vi "Test_Get MetaData.vi"() -> ()   [LabVIEW 2020]
uses:
  Measurement_client/RPC Messages/ni_measurements_v1_GetMetadataResponse.ctl
  Measurement_client/RPC Messages/ni_measurements_v1_MeasurementDetails.ctl
  Measurement_client/RPC Messages/ni_measurements_v1_MeasurementParameters.ctl
  Measurement_client/RPC Messages/ni_measurements_v1_ConfigurationParameter.ctl
  Measurement_client/RPC Messages/google_protobuf_Any.ctl
  Measurement_client/RPC Messages/ni_measurements_v1_Output.ctl
  Measurement_client/RPC Messages/ni_measurements_v1_UserInterfaceDetails.ctl
  Measurement_client/RPC Messages/ni_measurements_v1_GetMetadataRequest.ctl
  Measurement_client/Measurement_client.lvlib
panel:
  out "Response Data":T1
  in  "address":string
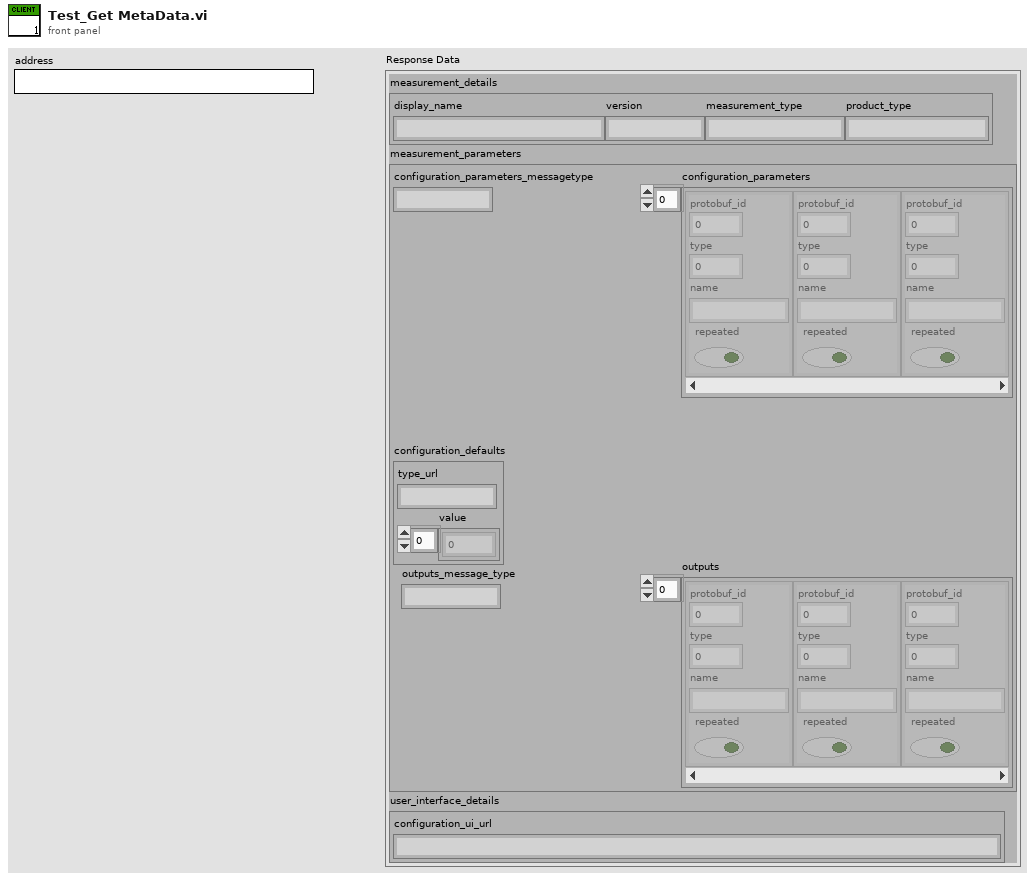
[diagram p1: front panel]
types:
  T1 = typedef "Measurement_client.lvlib/ni_measurements_v1_GetMetadataResponse.ctl" = cluster{"measurement_details":T2, "measurement_parameters":T3, "user_interface_details":T7}
  T2 = typedef "Measurement_client.lvlib/ni_measurements_v1_MeasurementDetails.ctl" = cluster{"display_name":string, "version":string, "measurement_type":string, "product_type":string}
  T3 = typedef "Measurement_client.lvlib/ni_measurements_v1_MeasurementParameters.ctl" = cluster{"configuration_parameters_messagetype":string, "configuration_parameters":T4[], "configuration_defaults":T5, "outputs_message_type":string, "outputs":T6[]}
  T4 = typedef "Measurement_client.lvlib/ni_measurements_v1_ConfigurationParameter.ctl" = cluster{"protobuf_id":u32, "type":i32, "name":string, "repeated":bool}
  T5 = typedef "Measurement_client.lvlib/google_protobuf_Any.ctl" = cluster{"type_url":string, "value":u8[]}
  T6 = typedef "Measurement_client.lvlib/ni_measurements_v1_Output.ctl" = cluster{"protobuf_id":u32, "type":i32, "name":string, "repeated":bool}
  T7 = typedef "Measurement_client.lvlib/ni_measurements_v1_UserInterfaceDetails.ctl" = cluster{"configuration_ui_url":string}
  T8 = typedef "Measurement_client.lvlib/ni_measurements_v1_GetMetadataRequest.ctl" = cluster{"void":string}
  T9 = typedef "gprc-lvsupport-release.lvlib/grpcId.ctl" = u64
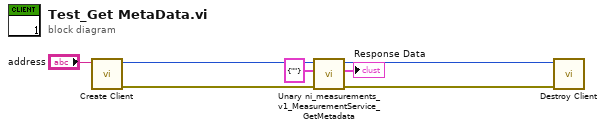
[diagram p0: block diagram]
diagram:
  n1 = call "Create Client.vi"("address"="address") -> ("error out"=w5:errorcluster, "gRPC ID Out"=w6:T9)  [unwired: 9 in]
  n2 = call "Unary ni_measurements_v1_MeasurementService_GetMetadata.vi"("error in"=w5, "Request Data"=T8 {"void"=""}, "gRPC ID"=w6) -> ("error out"=w3:errorcluster, "Response Data"=→"Response Data":T1, "gRPC ID out"=w4:T9)  [unwired: 6 in]
  n3 = call "Destroy Client.vi"("error in"=w3, "gRPC ID"=w4) -> ()  [unwired: 9 in, 1 out]
